vi "UART Read Benchmark.vi"() -> ()   [LabVIEW 2011]
uses:
  Private/Device/Device.lvlib
  Private/Type Defs/Interface.ctl
  LVH-LINX.lvlib
  <vilib>/ptbypt/NI_PtbyPt.lvlib
panel:
  in  "milliseconds to wait":u32
  in  "Stop Button":bool
  out "Data":string
  out "Bytes Availabe":u8
  out "Device Name":string
  out "Loop Rate":dbl(graph)
  out "Loop Time (ms)":i32
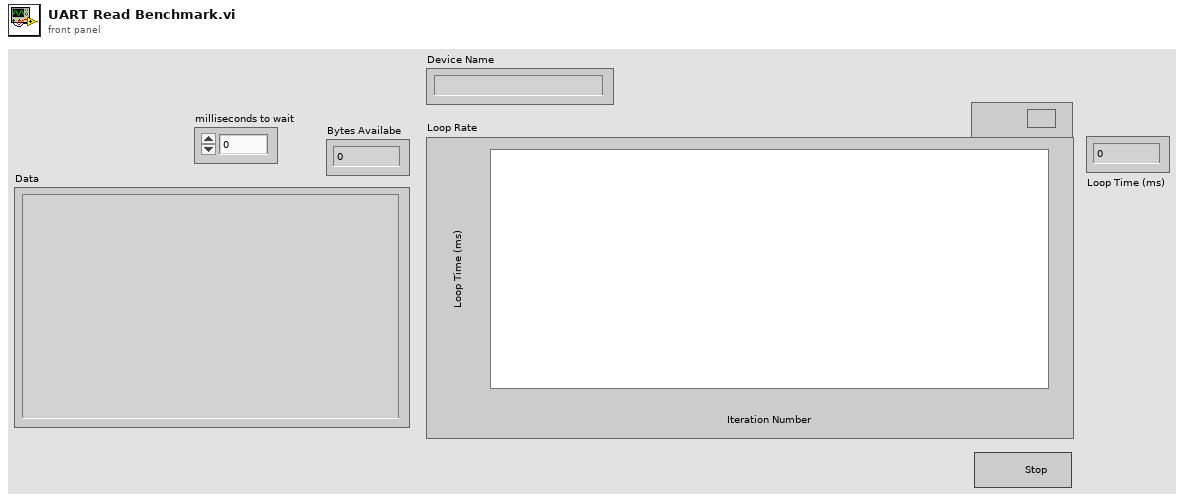
[diagram p1: front panel]
types:
  T1 = typedef "LVH-LINX.lvlib/Interface.ctl" = enum16{"Serial", "TCP"}
  T2 = typedef "LVH-LINX.lvlib/Device.lvlib/LINX Device Config.ctl" = cluster{"Interface":T1, "COM Port":refnum<visa-resource-name>, "TCP Configuration":T3, "Device Family":u8, "Device ID":u8, "Device Name":string, "TCP Ref":refnum<k5>, "Channels":T4}
  T3 = typedef "LVH-LINX.lvlib/Device.lvlib/TCP Config.ctl" = cluster{"IP Address":string, "Port":u16}
  T4 = typedef "LVH-LINX.lvlib/Channels.ctl" = cluster{"DI":u8[], "DO":u8[], "AI":u8[], "AO":u8[], "PWM":u8[], "QE":u8[], "UART":u8[], "I2C 2":u8[], "SPI":u8[], "CAN":u8[], "Servo":u8[], "AI Ref (V)":dbl, "AO Ref (V)":dbl, "AO Resolution (Bits)":u8}
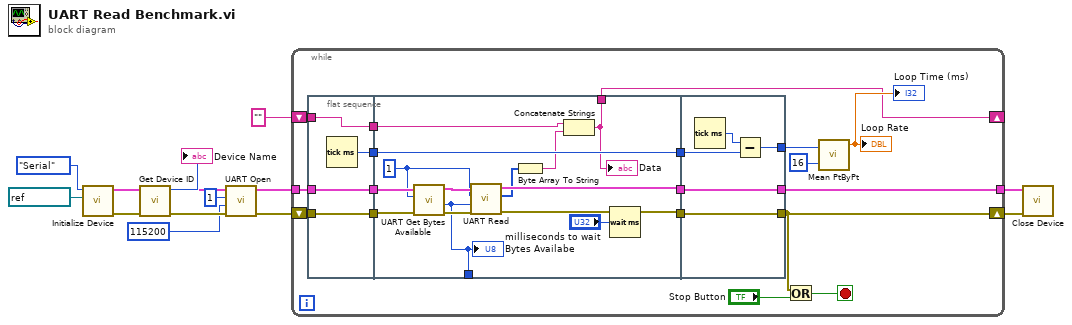
[diagram p0: block diagram]
diagram:
  n1 = call "Initialize Device.vi"("COM Port"=refnum<visa-resource-name> "COM5", "Interface"=Interface."Serial") -> ("Error Out"=w10:errorcluster, "LINX Device Config"=w11:T2)  [unwired: 8 in]
  n2 = call "Get Device ID.vi"("Error In"=w10, "LINX Device Config"=w11) -> ("Error Out"=w8:errorcluster, "Device Family"=→"Device Name":u8, "LINX Device Config"=w7:T2)  [unwired: 6 in, 1 out]
  n3 = call "UART Open.vi"("Error In"=w8, "Baud Rate (9600)"=u32 115200, "UART Channel"=u8 1, "LINX Device Config"=w7) -> ("Error Out"=w4:errorcluster, "LINX Device Config"=w3:T2)  [unwired: 6 in]
  n4 = while {
    shift-right: [w19] -> w12
    shift-left: w4 -> [w26]
    tunnel: w3 -> [w22]
    tunnel: [w21] -> w2
    shift-right: [w16] -> _
    shift-left: "" ("string") -> [w17]
    stop <- w32 stop-if-true
    n5 = flat-sequence {
      tunnel: [w36] -> w31
      tunnel: w26 -> [w35]
      tunnel: [w35] -> w25
      tunnel: [w34] -> w23
      tunnel: w22 -> [w34]
      tunnel: [w33] -> w18
      tunnel: w17 -> [w33]
      tunnel: w31 -> [w50]
      tunnel: [w50] -> w30
      tunnel: w25 -> [w46]
      tunnel: [w48] -> w24
      tunnel: w23 -> [w47]
      tunnel: [w49] -> w20
      tunnel: w18 -> [w40]
      tunnel: [w39] -> w16
      tunnel: [w38] -> _
      tunnel: w30 -> [w54]
      tunnel: [w53] -> w29
      tunnel: [w52] -> w19
      tunnel: w24 -> [w52]
      tunnel: [w51] -> w21
      tunnel: w20 -> [w51]
      frame #0 {
        n6 = Tick Count (ms)() -> (millisecond timer value=w36:u32)
      }
      frame #1 {
        w43 = u8 1 ("UART Channel")
        n7 = call "UART Get Bytes Available.vi"("Error In"=w46, "UART Channel"=w43, "LINX Device Config"=w47) -> ("Error Out"=w45:errorcluster, "Bytes Availabe"=w38:u8, "LINX Device Config"=w44:T2)  [unwired: 6 in]
        "Bytes Availabe" <- w38
        n8 = call "UART Read.vi"("Error In"=w45, "Num Bytes"=w38, "UART Channel"=w43, "LINX Device Config"=w44) -> ("Error Out"=w48:errorcluster, "Data"=w42:u8[], "LINX Device Config"=w49:T2)  [unwired: 5 in]
        n9 = Byte Array To String(unsigned byte array=w42) -> (string=w41:string)
        n10 = Concatenate Strings(w40, w41) -> (w39:string)
        "Data" <- w39
        n11 = Wait (ms)(milliseconds to wait="milliseconds to wait") -> ()  [unwired: 1 out]
      }
      frame #2 {
        n12 = Tick Count (ms)() -> (millisecond timer value=w55:u32)
        n13 = Subtract(x=w55, y=w54) -> (x-y=w53:u32)
      }
    }
    n14 = Or(x=w19, y="Stop Button") -> (x .or. y?=w32:bool)
    n15 = call <vilib>:"Mean PtByPt.vi"("x"=w29, "sample length"=16) -> ("mean"=→"Loop Rate" →"Loop Time (ms)":dbl)  [unwired: 2 in, 1 out]
  }
  n16 = call "Close Device.vi"("Error In"=w12, "LINX Device Config"=w2) -> ()  [unwired: 8 in, 2 out]
